vi "Read.vi"(11 "Register Select":bool) -> (3 "Data":u8)   [LabVIEW 2019, in "HD44780.lvlib"]
uses:
  HD44780.lvlib
  <vilib>/rvi/eio/common/nirviEmuTemplateMethod_errors.vi
  <vilib>/eio/EIONode/EIONode.xnode
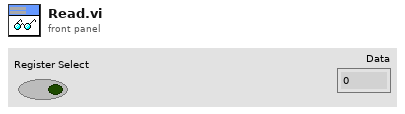
[diagram p1: front panel]
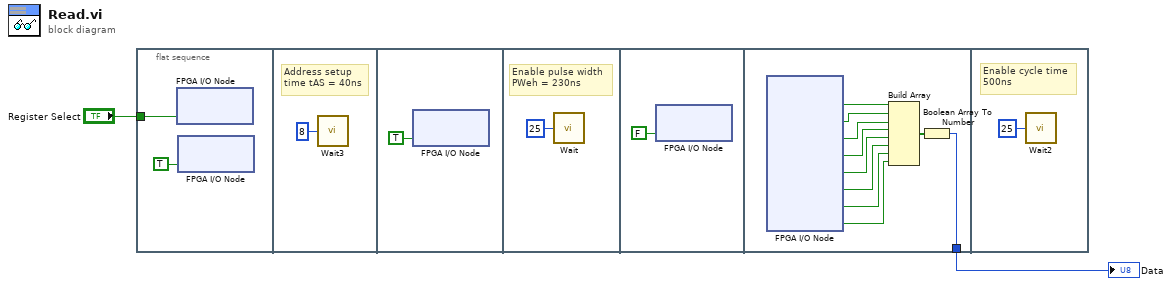
[diagram p0: block diagram]
diagram:
  n1 = flat-sequence {
    tunnel: "Register Select" -> [w3]
    tunnel: [w9] -> w2
    frame #0 {
      n2 = xnode "FPGA I/O Node"("RS"=w3) -> ()  [unwired: 1 in, 1 out]
      n3 = xnode "FPGA I/O Node"("RW"=TRUE) -> ()  [unwired: 1 in, 1 out]
    }
    frame #1 {
      # "Address setup\ntime tAS = 40ns"
      n4 = call "Wait3"("Count(Ticks)"=u8 8 ("Count(uSec)")) -> ()  [unwired: 1 out]
    }
    frame #2 {
      n5 = xnode "FPGA I/O Node"("E"=TRUE) -> ()  [unwired: 1 in, 1 out]
    }
    frame #3 {
      # "Enable pulse width\nPWeh = 230ns"
      n6 = call "Wait"("Count(Ticks)"=u8 25 ("Count(uSec)")) -> ()  [unwired: 1 out]
    }
    frame #4 {
      n7 = xnode "FPGA I/O Node"("E"=FALSE) -> ()  [unwired: 1 in, 1 out]
    }
    frame #5 {
      n8 = xnode "FPGA I/O Node"() -> ("DB0"=w10:bool, "DB1"=w11:bool, "DB2"=w12:bool, "DB3"=w13:bool, "DB4"=w14:bool, "DB5"=w15:bool, "DB6"=w16:bool, "DB7"=w17:bool)  [unwired: 8 in, 8 out]
      n9 = Build Array(w10, w11, w12, w13, w14, w15, w16, w17) -> (w18:bool[])
      n10 = Boolean Array To Number(Boolean array=w18) -> (number=w9:u8)
    }
    frame #6 {
      # "Enable cycle time\n500ns"
      n11 = call "Wait2"("Count(Ticks)"=u8 25 ("Count(uSec)")) -> ()  [unwired: 1 out]
    }
  }
  "Data" <- w2
